vi "Configure Waveform File Format.vi"(8 "error in (no error)":errorcluster, 10 "File Format (0: Internal)":i32(ring) items=["Internal", "Spreadsheet", "RF Baseband I&Q TIQ", "RF Baseband I&Q MATLAB"], 11 "VISA resource name":refnum<visa-resource-name>) -> (0 "error out":errorcluster, 3 "VISA resource name out":refnum<visa-resource-name>)   [LabVIEW 2016, in "Tektronix DPO MSO 2000 4000 Series.lvlib"]
doc: "Configures the waveform file format.\n\n<B>Notes:</B>\nThis VI is available for MDO4000 and MDO3000 Series only."
uses:
  Tektronix DPO MSO 2000 4000 Series.lvlib
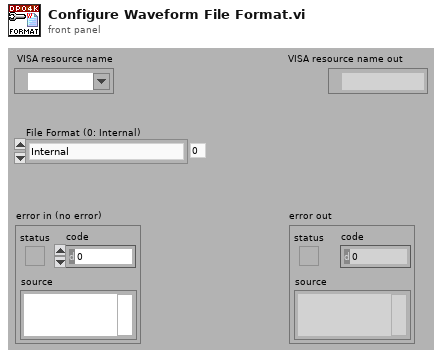
[diagram p1: front panel]
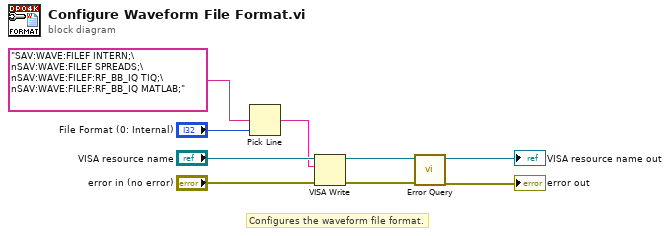
[diagram p0: block diagram]
diagram:
  # "Configures the waveform file format."
  n1 = Pick Line(multi-line string="SAV:WAVE:FILEF INTERN;\nSAV:WAVE:FILEF SPREADS;\nSAV:WAVE:FILEF:RF_BB_IQ TIQ;\nSAV:WAVE:FILEF:RF_BB_IQ MATLAB;", line index="File Format (0: Internal)") -> (output string=w2:string)  [unwired: 1 in]
  n2 = VISA Write(VISA resource name="VISA resource name", write buffer=w2, error in (no error)="error in (no error)") -> (VISA resource name out=w7:refnum<visa-resource-name>, error out=w6:errorcluster)  [unwired: 1 out]
  n3 = call "Error Query.vi"("error in (no error)"=w6, "VISA resource name"=w7) -> ("error out"=→"error out":errorcluster, "VISA resource name out"=→"VISA resource name out":refnum<visa-resource-name>)  [unwired: 6 in, 2 out]
